vi "FindLinearSlope.vi"(10 "length":i32, 11 "Array":dbl[](array[numeric])) -> (1 "slope":dbl, 2 "Best Linear Fit":dbl[](array[numeric]), 3 "Array out":i32[](array[numeric]))   [LabVIEW 2013, in "main.lvlib"]
uses:
  main.lvlib
  <vilib>/Analysis/NI_AALPro.lvlib
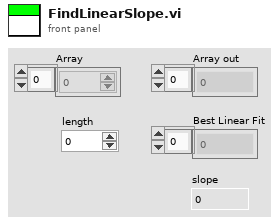
[diagram p1: front panel]
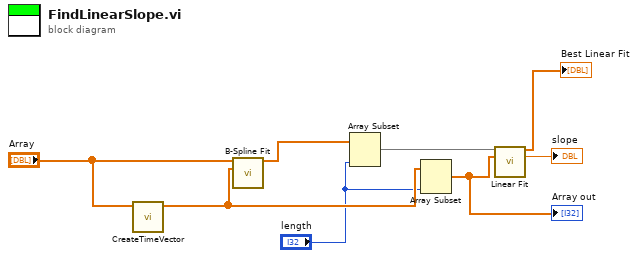
[diagram p0: block diagram]
diagram:
  n1 = call "CreateTimeVector.vi"("Array in"="Array") -> ("Array out"=w6:dbl[])  [unwired: 10 in]
  n2 = call <vilib>:"B-Spline Fit.vi"("Y"="Array", "X"=w6) -> ("Best BSpline Fit Y"=w7:dbl[])  [unwired: 10 in, 3 out]
  n3 = Array Subset(array=w7, length="length") -> (w3:dbl[])  [unwired: 1 in]
  n4 = Array Subset(array=w6, length="length") -> (w1:dbl[])  [unwired: 1 in]
  "Array out" <- w1
  n5 = call <vilib>:"Linear Fit.vi"("Y"=w3, "X"=w1) -> ("Best Linear Fit"=→"Best Linear Fit":dbl[], "slope"=→"slope":dbl)  [unwired: 9 in, 3 out]
